vi "Write Speaker Reference.vi"(8 "error in":errorcluster, 10 "SpkSw":refnum<class "Switch.lvclass">, 11 "PAS in":refnum<class "PAS.lvclass">) -> (0 "error out":errorcluster, 3 "PAS out":refnum<class "PAS.lvclass">)   [LabVIEW 2017, in "PAS Library.lvlib" / "PAS.lvclass"]
uses:
  PAS.lvclass
  Switch/Switch.lvclass
  PAS.lvclass/PAS.ctl
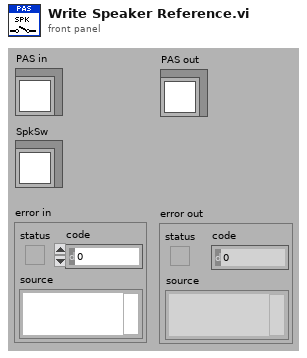
[diagram p1: front panel]
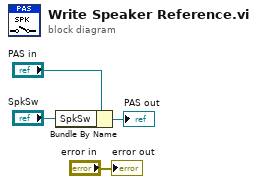
[diagram p0: block diagram]
diagram:
  n1 = Bundle By Name(cluster="PAS in", "SpkSw"="SpkSw") -> (→"PAS out":refnum<class "PAS.lvclass">)
  "error out" <- "error in"
